vi "FPGA_PPG_load_command.vi"(0 "resource_in":refnum<visa-resource-name>, 2 "command":string, 3 "mem_addr":u32, 5 "error in (no error)":errorcluster) -> (14 "resource_out":refnum<visa-resource-name>, 19 "error out":errorcluster)   [LabVIEW 2014, in "NI-FPGA_PPG_Driver.lvlib"]
doc: "Loads a single command to FPGA target specified by memory address. Also this VI can be used to replace one command.\n\nContact: Falk Ziegler, eMail: ziegler@physik.uni-greifswald.de"
uses:
  NI-FPGA_PPG_Driver.lvlib
  FPGA_PPG_error_type.ctl
  FPGA_PPG_action_type.ctl
  <vilib>/rvi/errors/niLvFpgaAdjustHostInterfaceError.vi
  <vilib>/rvi/interface/nirviReadWriteControl/nirviReadWriteControl.xnode
  FPGA_PPG_vi_ref.ctl
  FPGA Bitfiles/NI-FPGA-PPG.lvproj_PCI-7811R_FPGA_target_main.vi.lvbitx
  <vilib>/rvi/interface/nirviMethod/nirviMethod.xnode
  NiFpgaLv.dll
  <vilib>/FPGAPlugInAG/PCI-7811R/niLvFpga_WriteFifo_PCI-7811R.vi
  <vilib>/rvi/errors/niLvFpgaMergeErrorWithErrorCode.vi
panel:
  in  "errorCodes":T1
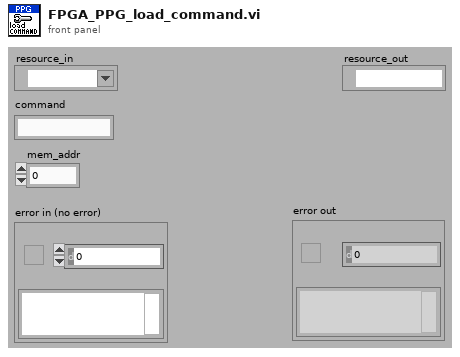
[diagram p1: front panel]
types:
  T1 = typedef "NI-FPGA_PPG_Driver.lvlib/FPGA_PPG_error_type.ctl" = enum16{"no error", "resource not initialized (no commands and invalid mem address)", "wrong memory address (address > Nof commands)", "invalid time value (probably too short)", "cannot start FPGA because one or more errors occured", "FIFO (internal) empty unexpectedly", "DMA FIFO (download from host) full unexpectedly", "checking number of commands: failed", "unknown error 8", "unknown error 9", "unknown error 10", "unknown error 11", "unknown error 12", "unknown error 13", "unknown error 14", "unknown error 15", "unknown error 16", "unknown error 17", "unknown error 18", "unknown error 19", "can't change state while pattern output is in progress"}
  T2 = typedef "NI-FPGA_PPG_Driver.lvlib/FPGA_PPG_action_type.ctl" = enum16{"GET", "SET", "REMOVE"}
  T3 = typedef "NI-FPGA_PPG_Driver.lvlib/FPGA_PPG_vi_ref.ctl" = refnum<k20>
  T4 = enum16{"idle", "reset", "query", "load", "run", "stopped"}
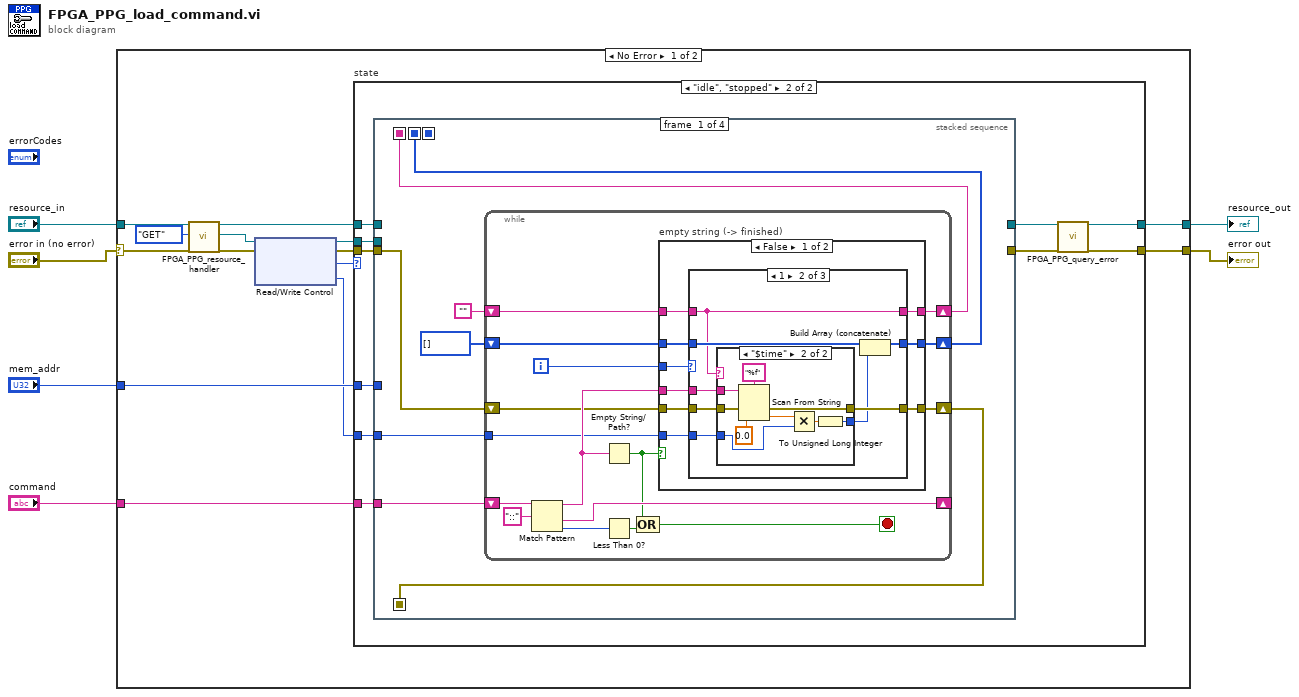
[diagram p0: block diagram]
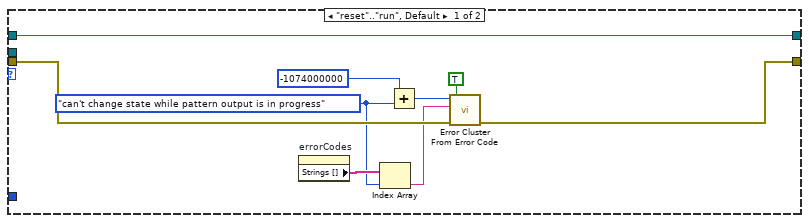
[diagram p2: hidden frame]
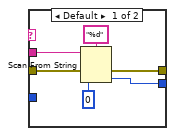
[diagram p4: hidden frame]
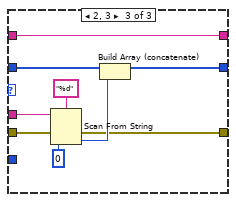
[diagram p5: hidden frame]
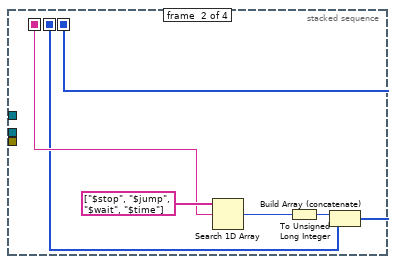
[diagram p7: hidden frame]
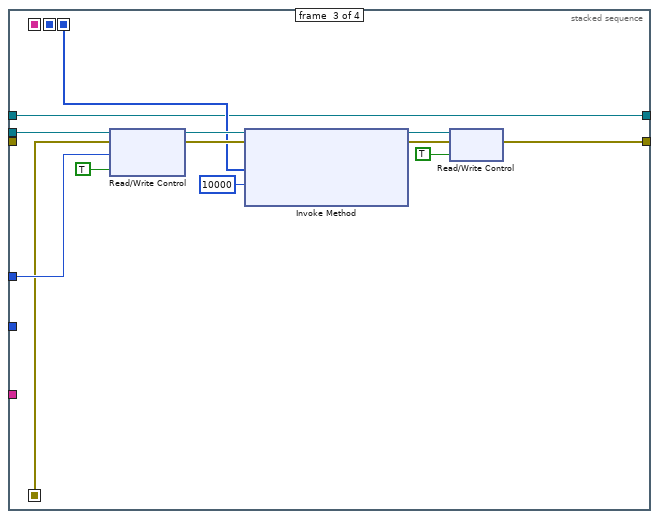
[diagram p8: hidden frame]
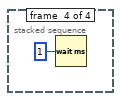
[diagram p9: hidden frame]
diagram:
  n1 = case shown="No Error" "error in (no error)" {
    selector: "error in (no error)" -> [w19 w132]
    tunnel: [w10 w132] -> w5
    tunnel: "resource_in" -> [w20 w131]
    tunnel: [w11 w131] -> w3
    tunnel: "command" -> [w16 _]
    tunnel: "mem_addr" -> [w13 _]
    frame No Error {
      n2 = call "FPGA_PPG_resource_handler.vi"("resource_in"=w20, "action"=FPGA_PPG_action_type."GET", "error in (no error)"=w19) -> ("resource_out"=w12:refnum<visa-resource-name>, "FPGA VI Reference Out"=w9:T3, "error out"=w18:errorcluster)  [unwired: 14 in]
      n3 = xnode "Read/Write Control"("FPGA VI Reference In"=w9, "error in"=w18) -> ("FPGA VI Reference Out"=w14:T3, "error out"=w15:errorcluster, "state"=w17:T4, "ticks_per_us"=w7:i32)
      n4 = case "state" shown="\"idle\", \"stopped\"" w17 {
        tunnel: w16 -> [_ w39]
        tunnel: w15 -> [w28 w38]
        tunnel: w14 -> [_ w37]
        tunnel: w13 -> [_ w36]
        tunnel: w12 -> [w29 w35]
        tunnel: [w29 w33] -> w11
        tunnel: [w27 w31] -> w10
        tunnel: w7 -> [_ w30]
        frame "reset".."run", Default {
          w21 = FPGA_PPG_error_type."can't change state while pattern output is in progress" ("errorCodes")
          n5 = property on="errorCodes" class="Enum (strict)"() -> ("Strings []"=w25:string[])  [unwired: 2 in, 2 out]
          n6 = Index Array(array=w25, index=w21) -> (element=w24:string)
          n7 = Add(x=-1074000000 ("error code (0)"), y=w21) -> (x+y=w22:i32)
          n8 = call <vilib>:"Error Cluster From Error Code.vi"("show call chain? (False)"=TRUE, "error in (no error)"=w28, "error message (\"\")"=w24, "error code (0)"=w22) -> ("error out"=w27:errorcluster)  [unwired: 5 in]
        }
        frame "idle", "stopped" {
          n9 = stacked-sequence {
            seq-local: [w43 _ _ _] -> [_ w115 _ _]
            seq-local: [w42 _ _ _] -> [_ _ w117 _]
            seq-local: [w41 _ _ _] -> [_ w113 _ _]
            seq-local: [_ w112 _ _] -> [_ _ w123 _]
            tunnel: w39 -> [w47 _ _ _]
            tunnel: w38 -> [w46 _ _ _]
            tunnel: w37 -> [_ _ w129 _]
            tunnel: w36 -> [_ _ w128 _]
            tunnel: w35 -> [_ _ w118 _]
            tunnel: [_ _ w118 _] -> w34
            tunnel: [_ _ w119 _] -> w32
            tunnel: w30 -> [w40 _ _ _]
            frame #0 {
              n10 = while {
                shift-right: [w60] -> _
                shift-left: w47 -> [w63]
                shift-right: [w57] -> w43
                shift-left: "" ("command") -> [w54]
                shift-right: [w56] -> w41
                shift-left: u32[] [] -> [w55]
                shift-right: [w53] -> w42
                shift-left: w46 -> [w52]
                tunnel: w40 -> [w48]
                i -> [w59]
                stop <- w49 stop-if-true
                n11 = Match Pattern(string=w63, regular expression="::") -> (before substring=w58:string, after substring=w60:string, offset past match=w61:i32)  [unwired: 1 in, 1 out]
                n12 = Empty String/Path?(string/path=w58) -> (empty?=w50:bool)
                n13 = Less Than 0?(x=w61) -> (x < 0?=w51:bool)
                n14 = Compound Arithmetic op=OR(w50, w51) -> (w49:bool)
                n15 = case "empty string (-> finished)" shown="False" w50 {
                  tunnel: w59 -> [w72 _]
                  tunnel: w58 -> [w71 _]
                  tunnel: [w70 w110] -> w57
                  tunnel: [w69 w109] -> w56
                  tunnel: w55 -> [w68 w109]
                  tunnel: w54 -> [w67 w110]
                  tunnel: [w66 w108] -> w53
                  tunnel: w52 -> [w65 w108]
                  tunnel: w48 -> [w64 _]
                  frame False {
                    n16 = case shown="1" w72 {
                      tunnel: w71 -> [w75 w83 w107]
                      tunnel: [w75 w77 w101] -> w70
                      tunnel: [w74 w82 w103] -> w69
                      tunnel: w68 -> [w74 w81 w102]
                      tunnel: w67 -> [_ w77 w101]
                      tunnel: [w73 w79 w100] -> w66
                      tunnel: w65 -> [w73 w80 w99]
                      tunnel: w64 -> [_ w76 _]
                      frame 0, Default {
                      }
                      frame 1 {
                        n17 = case shown="\"$time\"" w77 {
                          tunnel: w83 -> [w84 w98]
                          tunnel: w80 -> [w87 w95]
                          tunnel: [w86 w94] -> w79
                          tunnel: [w85 w91] -> w78
                          tunnel: w76 -> [_ w90]
                          frame Default {
                            n18 = Scan From String(format string="%d", input string=w84, error in=w87, default 1=u32 0 ("default value 1")) -> (error out=w86:errorcluster, output 1=w85:u32)  [unwired: 1 in, 2 out]
                          }
                          frame "$time" {
                            n19 = Scan From String(format string="%f", input string=w98, error in=w95, default 1=0.0 ("default value 1")) -> (error out=w94:errorcluster, output 1=w93:dbl)  [unwired: 1 in, 2 out]
                            n20 = Multiply(x=w93, y=w90) -> (x*y=w92:dbl)
                            n21 = To Unsigned Long Integer(number=w92) -> (unsigned 32bit integer=w91:u32)
                          }
                        }
                        n22 = Build Array (concatenate)(w81, w78) -> (w82:u32[])
                      }
                      frame 2, 3 {
                        n23 = Scan From String(format string="%d", input string=w107, error in=w99, default 1=u32 0 ("default value 1")) -> (error out=w100:errorcluster, output 1=w104:u32)  [unwired: 1 in, 2 out]
                        n24 = Build Array (concatenate)(w102, w104) -> (w103:u32[])
                      }
                    }
                  }
                  frame True {
                  }
                }
              }
            }
            frame #1 {
              n25 = Search 1D Array(1D array=string[] ["$stop", "$jump", "$wait", "$time"], element=w115) -> (index of element=w114:i32)  [unwired: 1 in]
              n26 = To Unsigned Long Integer(number=w114) -> (unsigned 32bit integer=w111:u32)
              n27 = Build Array (concatenate)(w111, w113) -> (w112:u32[])
            }
            frame #2 {
              n28 = xnode "Read/Write Control"("FPGA VI Reference In"=w129, "error in"=w117, "mem_addr"=w128, "replace"=TRUE) -> ("FPGA VI Reference Out"=w125:T3, "error out"=w124:errorcluster)
              n29 = xnode "Invoke Method"("FPGA VI Reference In"=w125, "error in"=w124, "Data"=w123, "Timeout (ms)"=10000) -> ("FPGA VI Reference Out"=w122:T3, "error out"=w121:errorcluster)  [unwired: 1 out]
              n30 = xnode "Read/Write Control"("FPGA VI Reference In"=w122, "error in"=w121, "load"=TRUE) -> ("error out"=w119:errorcluster)  [unwired: 1 out]
            }
            frame #3 {
              n31 = Wait (ms)(milliseconds to wait=u32 1) -> ()  [unwired: 1 out]
            }
          }
          n32 = call "FPGA_PPG_query_error.vi"("resource_in"=w34, "error in (no error)"=w32) -> ("resource_out"=w33:refnum<visa-resource-name>, "error out"=w31:errorcluster)  [unwired: 16 in]
        }
      }
    }
    frame Error {
    }
  }
  "error out" <- w5
  "resource_out" <- w3
